vi "encodeCluster.vi"(6 "MsgPack Config":T1={"Cluster Conversion"=enum."to array", "Enum Conversion"=enum."to uint", "Use ArrayType"=FALSE}, 8 "error in (no error)":errorcluster, 10 "Variant":variant) -> (0 "error out":errorcluster, 2 "Array":u8[](array[numeric]) format="%.0x")   [LabVIEW 2016, in "MsgPack.lvlib"]
uses:
  MsgPack.lvlib
  SubVis/msgpack_config.ctl
  SubVis/cluster_conversion.ctl
  SubVis/enum_conversion.ctl
  <vilib>/Utility/error.llb/Error Cluster From Error Code.vi
  <vilib>/ErrorRing/Error Ring.xnode
  <vilib>/Utility/Data Type/NI_Data Type.lvlib
panel:
  out "Element Names":string[](array[string])
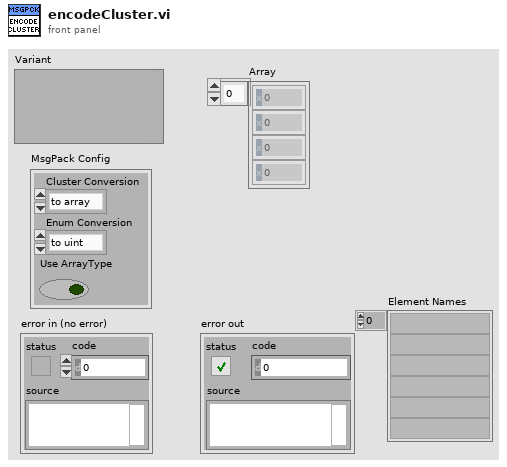
[diagram p1: front panel]
types:
  T1 = typedef "MsgPack.lvlib/msgpack_config.ctl" = cluster{"Cluster Conversion":T2, "Enum Conversion":T3, "Use ArrayType":bool}
  T2 = typedef "MsgPack.lvlib/cluster_conversion.ctl" = enum16{"to map", "to array"}
  T3 = typedef "MsgPack.lvlib/enum_conversion.ctl" = enum16{"to uint", "to string"}
  T4 = typedef "NI_Data Type.lvlib/Data Type.ctl" = enum8{"Invalid Type", "Void", "I8", "I16", "I32", "I64", "U8", "U16", "U32", "U64", "Single Float", "Double Float", "Extended Float", "Single Complex", "Double Complex", "Extended Complex", "Enum U8", "Enum U16", "Enum U32", "Enum U64", "Single Float With Unit", "Double Float With Unit", "Extended Float With Unit", "Single Complex with Unit", "Double Complex with Unit", "Extended Complex with Unit", "Boolean", "String", "Path", "Picture", "Tag", "Array", "Cluster", "Variant", "LV Variant", "Waveform", "Timestamp", "Digital Waveform", "Digital Data", "ExpressData", "Refnum", "External Data", "VI", "Poly VI", "LabVIEW Class Instance", "Fixed Point"}
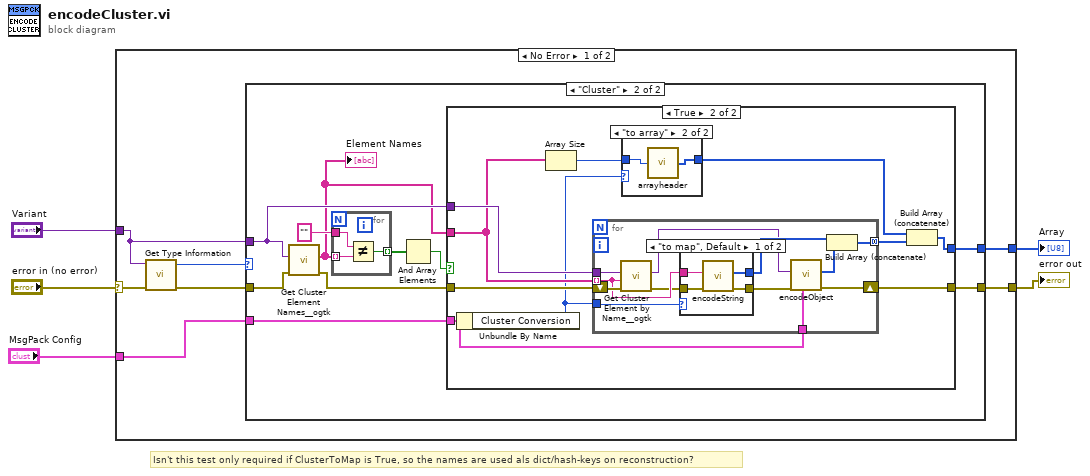
[diagram p0: block diagram]
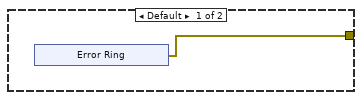
[diagram p2: hidden frame]
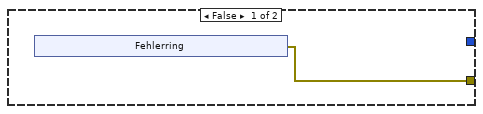
[diagram p3: hidden frame]
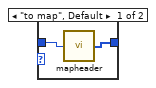
[diagram p4: hidden frame]
diagram:
  # "Isn't this test only required if ClusterToMap is True, so the names are used als dict/hash-keys on reconstruction?"
  n1 = case shown="No Error" "error in (no error)" {
    selector: "error in (no error)" -> [w7 w69]
    tunnel: [w10 _] -> w5
    tunnel: [w9 w69] -> w4
    tunnel: "Variant" -> [w8 _]
    tunnel: "MsgPack Config" -> [w6 _]
    frame No Error {
      n2 = call <vilib>:"Get Type Information.vi"("error in (no error)"=w7, "Variant"=w8) -> ("error out"=w11:errorcluster, "Type"=w12:T4)  [unwired: 5 in, 3 out]
      n3 = case shown="\"Cluster\"" w12 {
        tunnel: w11 -> [_ w26]
        tunnel: w8 -> [_ w21]
        tunnel: [_ w28] -> w10
        tunnel: [w13 w27] -> w9
        tunnel: w6 -> [_ w19]
        frame Default {
          n4 = xnode "Error Ring"() -> ("error out"=w13:errorcluster)
        }
        frame "Cluster" {
          n5 = call <userlib>:"Get Cluster Element Names__ogtk.vi"("error in (no error)"=w26, "Cluster"=w21) -> ("error out"=w25:errorcluster, "Element Names"=w20:string[])  [unwired: 8 in]
          "Element Names" <- w20
          n6 = for {
            tunnel: w20 -> [w68] mode=indexing
            tunnel: "" ("x") -> [w67]
            tunnel: [w66] -> w23 mode=indexing
            n7 = Not Equal?(x=w67, y=w68) -> (x != y?=w66:bool)
          }
          n8 = And Array Elements(Boolean array=w23) -> (logical AND=w22:bool)
          n9 = case shown="True" w22 {
            tunnel: [_ w44] -> w28
            tunnel: [w29 w37] -> w27
            tunnel: w25 -> [_ w39]
            tunnel: w21 -> [_ w41]
            tunnel: w20 -> [_ w40]
            tunnel: w19 -> [_ w36]
            frame False {
              n10 = xnode "Fehlerring"() -> ("error out"=w29:errorcluster)
            }
            frame True {
              n11 = Unbundle By Name(w36) -> ("Cluster Conversion"=w35:T2)
              n12 = Array Size(array=w40) -> (size(s)=w43:i32)
              n13 = for {
                tunnel: w40 -> [w58] mode=indexing
                shift-right: [w53] -> w37
                shift-left: w39 -> [w60]
                tunnel: w41 -> [w59]
                tunnel: [w50] -> w38 mode=concatenating
                tunnel: w35 -> [w52]
                tunnel: w36 -> [w49]
                n14 = call <userlib>:"Get Cluster Element by Name__ogtk.vi"("error in (no error)"=w60, "Element Name"=w58, "Cluster"=w59) -> ("error out"=w57:errorcluster, "VElement"=w54:variant)  [unwired: 6 in, 1 out]
                n15 = case shown="\"to map\", Default" w52 {
                  tunnel: w58 -> [w64 _]
                  tunnel: w57 -> [w63 w65]
                  tunnel: [w62 w65] -> w56
                  tunnel: [w61 _] -> w55
                  frame "to map", Default {
                    n16 = call "encodeString.vi"("error in (no error)"=w63, "Variant"=w64) -> ("error out"=w62:errorcluster, "Array"=w61:u8[])  [unwired: 8 in]
                  }
                  frame "to array" {
                  }
                }
                n17 = call "encodeObject.vi"("MsgPack Config"=w49, "error in (no error)"=w56, "Variant"=w54) -> ("error out"=w53:errorcluster, "Array"=w51:u8[])  [unwired: 7 in]
                n18 = Build Array (concatenate)(w55, w51) -> (w50:u8[])
              }
              n19 = case shown="\"to array\"" w35 {
                tunnel: w43 -> [w46 w48]
                tunnel: [w45 w47] -> w42
                frame "to map", Default {
                  n20 = call "mapheader.vi"("Number of Elements"=w46) -> ("header"=w45:u8[])
                }
                frame "to array" {
                  n21 = call "arrayheader.vi"("Number of Elements"=w48) -> ("header"=w47:u8[])
                }
              }
              n22 = Build Array (concatenate)(w42, w38) -> (w44:u8[])
            }
          }
        }
      }
    }
    frame Error {
    }
  }
  "Array" <- w5
  "error out" <- w4
